vi "datadictionary.vi"(11 "data dictionary in":refnum<class "data dictionary.lvclass">) -> (2 "Value String":string, 3 "Boolean":bool)   [LabVIEW 2013, in "tag bus.lvlib" / "data dictionary.lvclass"]
uses:
  dictionary/data dictionary.lvclass
  tag/Data Type.ctl
  tag/tag descriptor.lvclass
panel:
  out "data type":T1
  out "index":i32
  in  "name":string
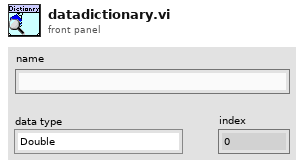
[diagram p1: front panel]
types:
  T1 = typedef "tag bus.lvlib/tag descriptor.lvclass/Data Type.ctl" = enum16{"Double", "Single", "I64", "I32", "I16", "I8", "U64", "U32", "U16", "U8", "Boolean", "String", "Array of Double", "Array of Single", "Array of I64", "Array of I32", "Array of I16", "Array of I8", "Array of U64", "Array of U32", "Array of U16", "Array of U8", "Array of Boolean", "Array of String"}
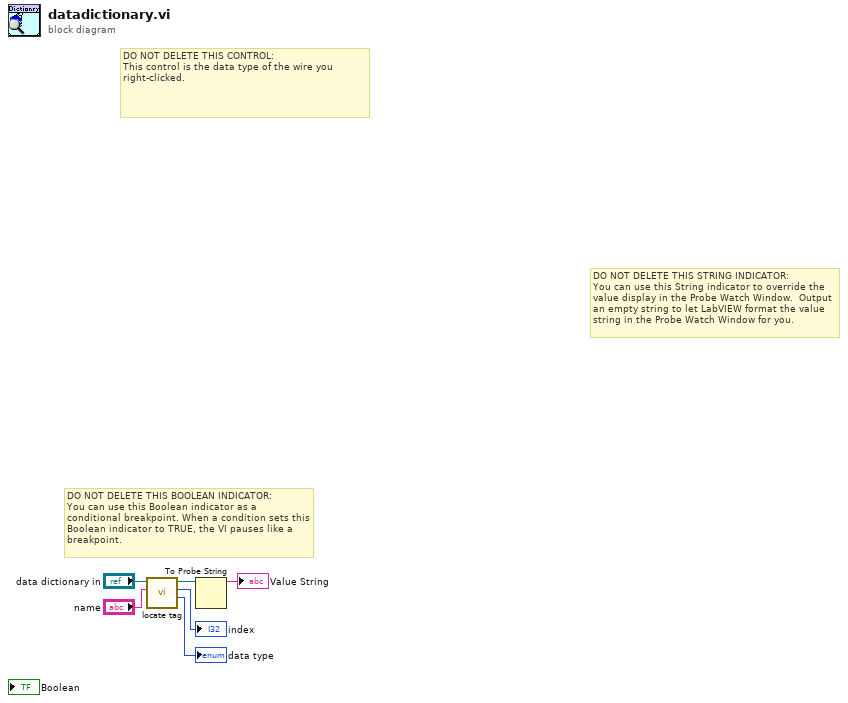
[diagram p0: block diagram]
diagram:
  # "DO NOT DELETE THIS STRING INDICATOR: \nYou can use this String indicator to override the value display in the Probe Watch Window.  Output an empty string to let LabVIEW format the value string in the Probe Watch Window for you."
  # "DO NOT DELETE THIS BOOLEAN INDICATOR: \nYou can use this Boolean indicator as a conditional breakpoint. When a condition sets this Boolean indicator to TRUE, the VI pauses like a breakpoint."
  # "DO NOT DELETE THIS CONTROL: \nThis control is the data type of the wire you right-clicked."
  n1 = call "locate tag.vi"("name"="name", "data dictionary in"="data dictionary in") -> ("data type"=→"data type":T1, "index"=→"index":i32, "data dictionary out"=w4:refnum<class "data dictionary.lvclass">)  [unwired: 6 in, 1 out]
  n2 = To Probe String(7:w4) -> (3:→"Value String":string)  [unwired: 2 in, 1 out]
